vi "Variation Band.vi"(11 "Data":dbl[](array[numeric])) -> ()   [LabVIEW 2016]
uses:
  <vilib>/Analysis/NI_AALBase.lvlib
  <vilib>/gmath/NI_Gmath.lvlib
panel:
  out "Waveform Graph":waveform(dbl)[](graph)
  out "Min":dbl[](array[numeric])
  out "Max":dbl[](array[numeric])
  in  "Window width":i32=100
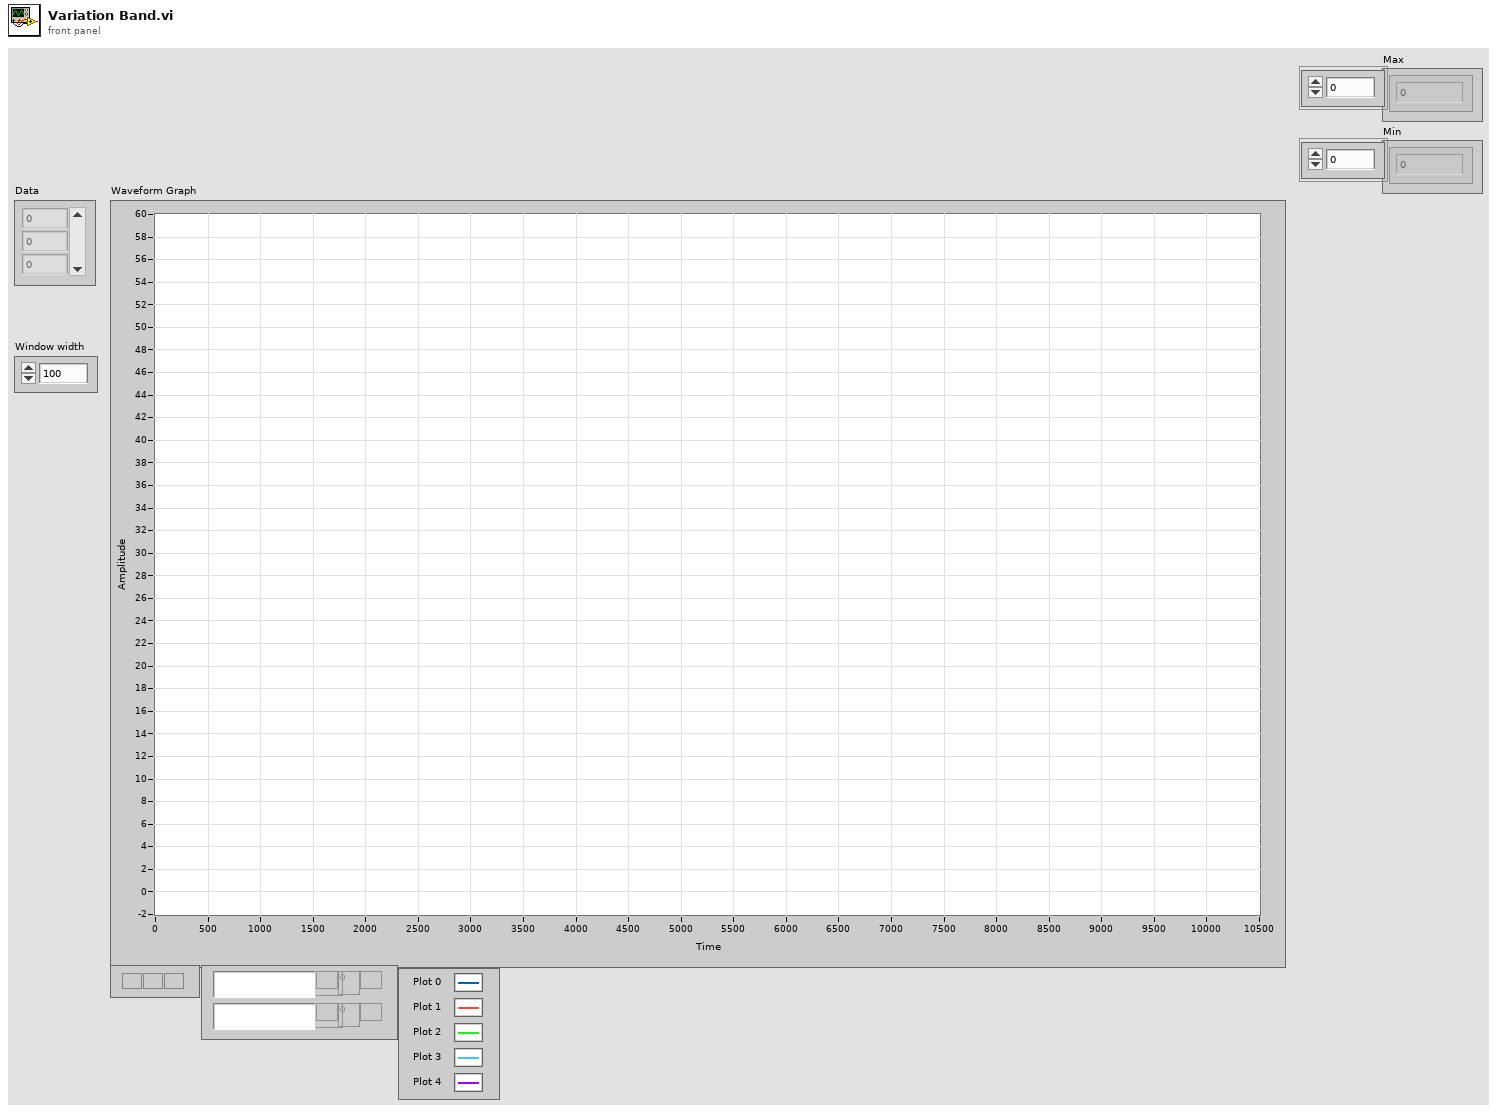
[diagram p1: front panel]
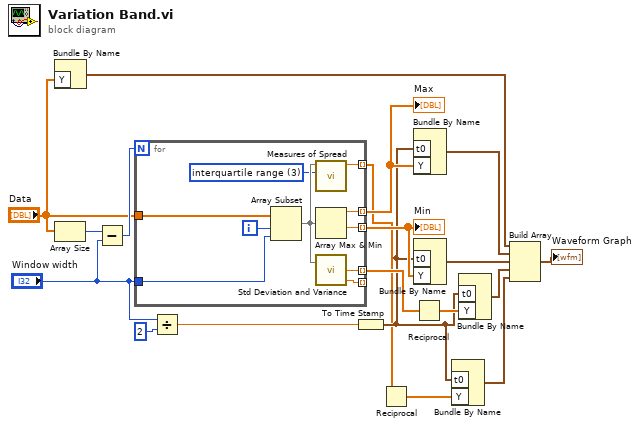
[diagram p0: block diagram]
diagram:
  n1 = Bundle By Name("Y"="Data") -> (w16:waveform(dbl))  [unwired: 1 in]
  n2 = Array Size(array="Data") -> (size(s)=w19:i32)
  n3 = Subtract(x=w19, y="Window width") -> (x-y=w18:i32)
  n4 = for {
    N: w18 -> [_]
    tunnel: "Data" -> [w29]
    tunnel: "Window width" -> [w27]
    tunnel: [w26] -> w11 mode=indexing
    tunnel: [w25] -> w12 mode=indexing
    tunnel: [w24] -> w5 mode=indexing
    tunnel: [w23] -> _ mode=indexing
    tunnel: [w20] -> w3 mode=indexing
    i -> [w28]
    w21 = 3 items=["standard deviation", "range", "mean absolute deviation", "interquartile range"] ("type")
    n5 = Array Subset(array=w29, index=w28, length=w27) -> (w22:dbl[])
    n6 = call <vilib>:"Measures of Spread.vi"("type"=w21, "x array"=w22) -> ("spread value"=w20:dbl)  [unwired: 8 in, 1 out]
    n7 = Array Max & Min(array=w22) -> (max value=w25:dbl, min value=w26:dbl)  [unwired: 2 out]
    n8 = call <vilib>:"Std Deviation and Variance.vi"("X"=w22) -> ("standard deviation"=w24:dbl, "variance"=w23:dbl)  [unwired: 1 in, 1 out]
  }
  "Max" <- w12
  "Min" <- w11
  n9 = Divide(x="Window width", y=2) -> (x/y=w13:dbl)
  n10 = To Time Stamp(1:w13) -> (0:w4:timestamp)
  n11 = Reciprocal(x=w3) -> (1/x=w1:dbl[])
  n12 = Bundle By Name("t0"=w4, "Y"=w12) -> (w10:waveform(dbl))  [unwired: 1 in]
  n13 = Bundle By Name("t0"=w4, "Y"=w11) -> (w9:waveform(dbl))  [unwired: 1 in]
  n14 = Reciprocal(x=w5) -> (1/x=w6:dbl[])
  n15 = Bundle By Name("t0"=w4, "Y"=w1) -> (w2:waveform(dbl))  [unwired: 1 in]
  n16 = Bundle By Name("t0"=w4, "Y"=w6) -> (w7:waveform(dbl))  [unwired: 1 in]
  n17 = Build Array(w16, w10, w9, w7, w2) -> (→"Waveform Graph":waveform(dbl)[])
